vi "Pack.vi"(11 "Packet":T1) -> (3 "ClusterMessagePacket out":refnum<class "ClusterMessagePacket.lvclass">)   [LabVIEW 2020, in "Network Messenger.lvlib" / "ClusterMessagePacket.lvclass"]
uses:
  <vilib>/gpm_packages/@cs/Network-interface/Source/Network Messenger/ClusterMessagePacket/ClusterMessagePacket.lvclass
  <vilib>/gpm_packages/@cs/Network-interface/Source/Network Messenger/Types/Message Packet.ctl
  <vilib>/gpm_packages/@cs/Network-interface/Source/Network Messenger/ClusterMessagePacket/ClusterMessagePacket.lvclass/ClusterMessagePacket.ctl
  <vilib>/gpm_packages/@cs/Network-interface/Source/Network Messenger/Network Messenger.lvlib
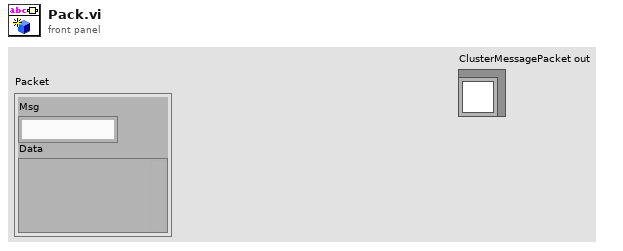
[diagram p1: front panel]
types:
  T1 = typedef "Network Messenger.lvlib/Message Packet.ctl" = cluster{"Msg":string, "Data":variant}
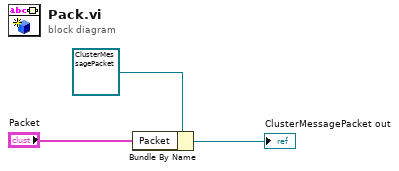
[diagram p0: block diagram]
diagram:
  n1 = Bundle By Name(cluster=refnum<class "ClusterMessagePacket.lvclass"> refnum ("ClusterMessagePacket in"), "Packet"="Packet") -> (→"ClusterMessagePacket out":refnum<class "ClusterMessagePacket.lvclass">)
